vi "Init Settings.vi"(8 "error in":errorcluster, 11 "Analog-Output in":refnum<class "Analog-Output.lvclass">) -> (0 "error out":errorcluster, 3 "Analog-Output out":refnum<class "Analog-Output.lvclass">)   [LabVIEW 2019, in "Analog-Output.lvlib" / "Analog-Output.lvclass"]
uses:
  Library/Analog-Output.lvclass
  Library/Analog-Output.lvclass/Analog-Output.ctl
  Custom Controls/Settings.ctl
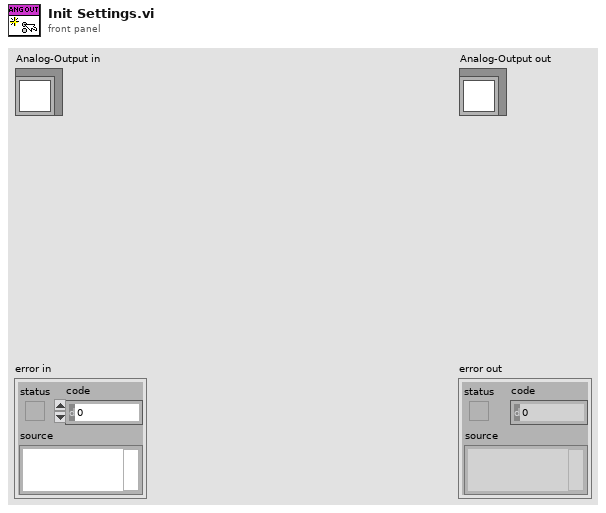
[diagram p1: front panel]
types:
  T1 = typedef "Analog-Output.lvlib/Analog-Output.lvclass/Settings.ctl" = cluster{"Voltage":dbl}
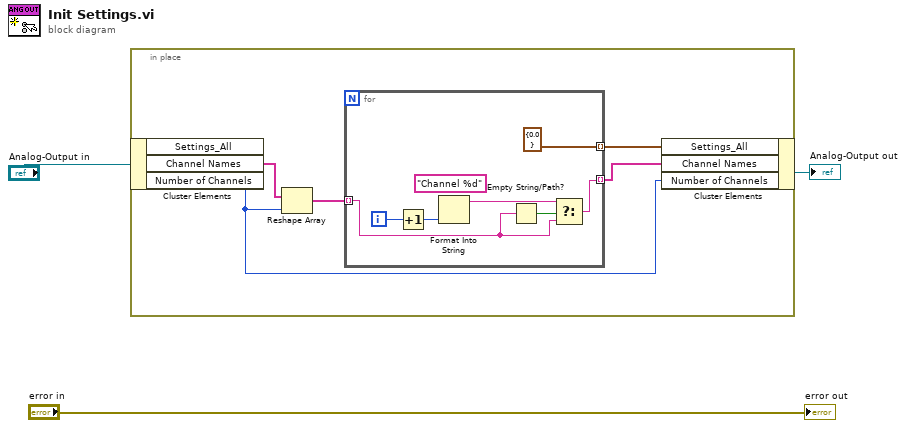
[diagram p0: block diagram]
diagram:
  n1 = in-place {
    n2 = in-place-cluster #1("Analog-Output in") -> ("Channel Names"=w8:string[], "Number of Channels"=w4:i32)  [unwired: 1 out]
    n3 = Reshape Array(w8, w4) -> (w7:string[])
    n4 = for {
      tunnel: w7 -> [w11] mode=indexing
      tunnel: [T1 {"Voltage"=0.0} ("Settings")] -> w6 mode=indexing
      tunnel: [w9] -> w5 mode=indexing
      i -> [w10]
      (unwired) "Channel %d" ("format string")
      n5 = Increment(x=w10) -> (x+1=w13:i32)
      n6 = Format Into String(w13) -> (resulting string=w12:string)  [unwired: 3 in, 1 out]
      n7 = Empty String/Path?(string/path=w11) -> (empty?=w14:bool)
      n8 = Select(t=w12, s=w14, f=w11) -> (s? t:f=w9:string)
    }
    n9 = in-place-cluster #1("Settings_All"=w6, "Channel Names"=w5, "Number of Channels"=w4) -> (→"Analog-Output out":refnum<class "Analog-Output.lvclass">)
  }
  "error out" <- "error in"
